vi "Get Nested Tag.vi"(8 "error in (no error)":errorcluster, 10 "Path":cluster{"Tag ID / Name":variant, "Index":i32}[](array[cluster]), 11 "Raw Message in":refnum<class "Raw Message.lvclass">) -> (0 "error out":errorcluster, 2 "Tag":refnum<class "Basic Type.lvclass">, 3 "Nested Message":refnum<class "Raw Message.lvclass">)   [LabVIEW 2020, in "Protobuf RAW.lvlib" / "Raw Message.lvclass"]
uses:
  Raw Message.lvclass
  Raw Message.lvclass/Raw Message.ctl
  <vilib>/Utility/Data Type/Get Type Information.vi
  Tag/Basic Type.lvclass
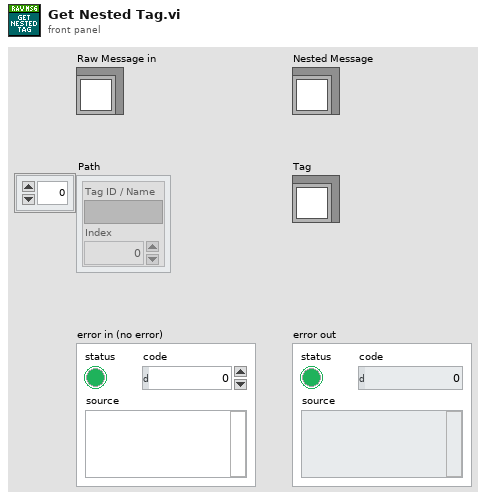
[diagram p1: front panel]
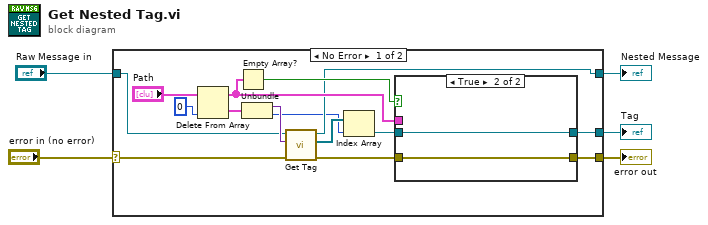
[diagram p0: block diagram]
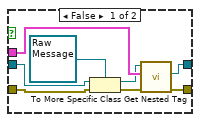
[diagram p2: hidden frame]
diagram:
  n1 = case shown="No Error" "error in (no error)" {
    selector: "error in (no error)" -> [w15 w31]
    tunnel: [w6 w31] -> w5
    tunnel: [w12 _] -> w4
    tunnel: "Raw Message in" -> [w13 _]
    tunnel: [w9 _] -> w1
    frame No Error {
      n2 = Delete From Array(array="Path", index=0) -> (deleted portion=w17:cluster{"Tag ID / Name":variant, "Index":i32}, array with subset deleted=w16:cluster{"Tag ID / Name":variant, "Index":i32}[])  [unwired: 1 in]
      n3 = Empty Array?(array=w16) -> (empty?=w18:bool)
      n4 = Unbundle(w17) -> ("Tag ID / Name"=w14:variant, "Index"=w10:i32)
      n5 = call "Get Tag.vi"("error in (no error)"=w15, "ID / Name"=w14, "Raw Message in"=w13) -> ("error out"=w7:errorcluster, "Tags"=w11:refnum<class "Basic Type.lvclass">[], "Raw Message out"=w12:refnum<class "Raw Message.lvclass">)  [unwired: 6 in]
      n6 = Index Array(array=w11, index=w10) -> (element=w8:refnum<class "Basic Type.lvclass">)
      n7 = case shown="True" w18 {
        tunnel: w16 -> [w28 _]
        tunnel: [w22 w30] -> w9
        tunnel: w8 -> [w27 w30]
        tunnel: w7 -> [w26 w29]
        tunnel: [w21 w29] -> w6
        frame False {
          n8 = To More Specific Class(target class=refnum<class "Raw Message.lvclass"> refnum ("Protobuf RAW.lvlib:Raw Message.lvclass"), reference=w27, error in=w26) -> (specific class reference=w23:refnum<class "Raw Message.lvclass">, error out=w25:errorcluster)
          n9 = call "Get Nested Tag.vi"("error in (no error)"=w25, "Path"=w28, "Raw Message in"=w23) -> ("error out"=w21:errorcluster, "Tag"=w22:refnum<class "Basic Type.lvclass">)  [unwired: 6 in, 1 out]
        }
        frame True {
        }
      }
    }
    frame Error {
    }
  }
  "error out" <- w5
  "Nested Message" <- w4
  "Tag" <- w1
